vi "Atmospheric Constants.vi"() -> ()   [LabVIEW 2016, in "Atmospheric Library.lvlib"]
uses:
  Atmospheric Library.lvlib
panel:
  in  "A (molecules/mol)":dbl=6.0225e+23
  in  "Torr->mb":sgl=1.33322
  in  "g (m/s2)":dbl=9.807
  in  "Rd (J/(kg K)":dbl=286.9
  in  "R (J/(mol K)":dbl=8.314472
  in  "Nref (m-3)":dbl=2.50362e+25
  in  "PSI->mb":sgl=68.94757
  in  "c (m/s)":dbl=299792458.0
  in  "e0 (Farad/m)":dbl=8.85e-12
  in  "Mw (kg/kmol)":dbl=18.02
  in  "Ma (kg/kmol)":dbl=28.97
  in  "e (C)":dbl=1.60217646e-19
  in  "k (J/K)":dbl=1.3806503e-23
  in  "P0 (mb)":sgl=1013.25
  in  "Tn (K)":dbl=273.15
  in  "T0 (K)":sgl=293.15
  in  "l0 (mm)":dbl=0.066
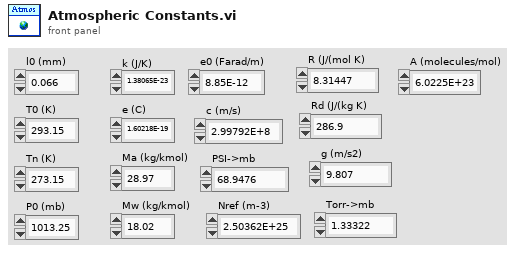
[diagram p1: front panel]
diagram:
